vi "GT 2D Compare Status.vi"(0 "cardNum":i16, 1 "chn":i16, 2 "pStatus":i16, 3 "pCount":i32, 4 "pFifo":i16, 5 "pFifoCount":i16, 6 "pBufCount":i16, 7 "error in (no error)":errorcluster caption="错误输入（无错误）") -> (20 "function return":i16, 22 "pStatus out":i16, 23 "pCount out":i32, 24 "pFifo out":i16, 25 "pFifoCount out":i16, 26 "pBufCount out":i16, 27 "error out":errorcluster caption="错误输出")   [LabVIEW 2020, in "gts.lvlib"]
doc: "GT_API GT_2DCompareStatus(short cardNum,short chn,short *pStatus,long *pCount,short *pFifo,short *pFifoCount,short *pBufCount =NULL);"
uses:
  gts.lvlib
  dll/32bit/multi_card/gts.dll
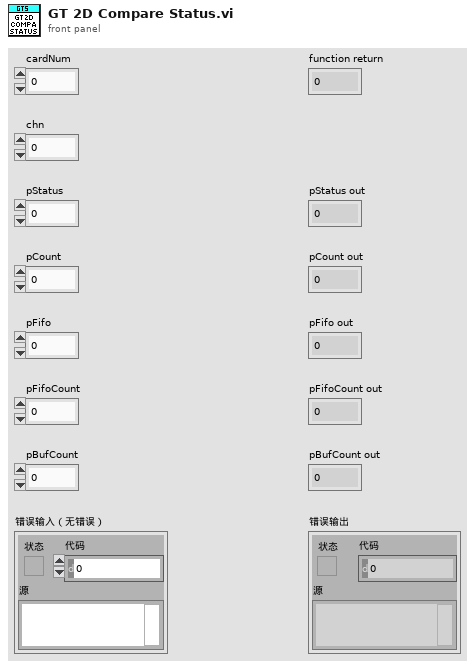
[diagram p1: front panel]
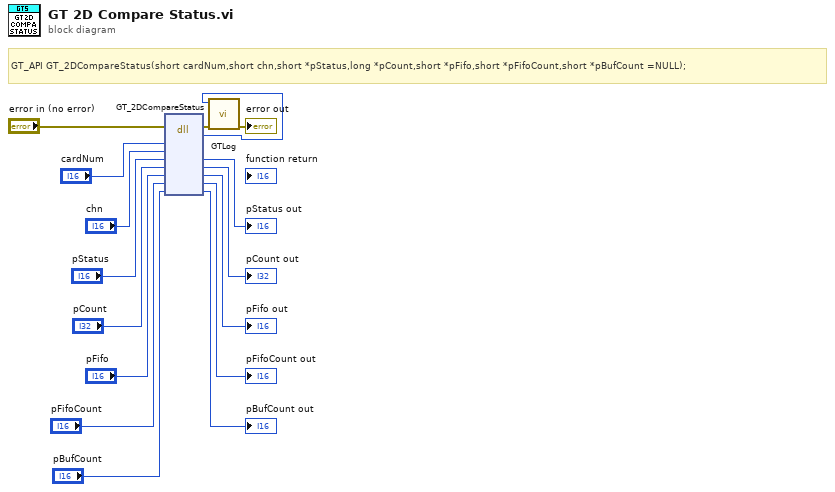
[diagram p0: block diagram]
diagram:
  # "GT_API GT_2DCompareStatus(short cardNum,short chn,short *pStatus,long *pCount,short *pFifo,short *pFifoCount,short *pBufCount =NULL);"
  n1 = dll-call lib="D:/Git/GoogolCard/dll/32bit/multi_card/gts.dll" fn="GT_2DCompareStatus"(error in="error in (no error)", "cardNum"="cardNum", "chn"="chn", "pStatus"="pStatus", "pCount"="pCount", "pFifo"="pFifo", "pFifoCount"="pFifoCount", "pBufCount"="pBufCount") -> (error out=w3:errorcluster, "返回类型"=w1:i16, "pStatus"=→"pStatus out":i16, "pCount"=→"pCount out":i32, "pFifo"=→"pFifo out":i16, "pFifoCount"=→"pFifoCount out":i16, "pBufCount"=→"pBufCount out":i16)  [unwired: 4 in, 1 out]
  n2 = call "GTLog.vi"("error in (no error)"=w3, "Numeric"=w1) -> ("error out"=→"error out":errorcluster)  [unwired: 9 in]
